vi "GPS (11.25).vi"() -> ()   [LabVIEW 2018]
uses:
  <vilib>/Instr/_visa.llb/VISA Configure Serial Port (Instr).vi
  <vilib>/Utility/file.llb/Read Delimited Spreadsheet (DBL).vi
panel:
  in  "로깅 정지":bool
  in  "Logging 저장위치":path
  in  "Logging On/Off":bool
  out "in out 상태":bool
  out "직선":bool
  out "곡선":bool
  out "주행완료":bool
  out "count":dbl
  out "설정 반지름":dbl
  out "중간":bool
  out "in":bool
  out "out":bool
  out "코스 판별":dbl(slide) scale=0.0..1.0
  out "out 근접":dbl
  out "in 근접":dbl
  out "RDDF Y_in":dbl[](array[numeric]) format="%#_10g"
  out "RDDF X_in":dbl[](array[numeric]) format="%#_10g"
  out "RDDF Y_out":dbl[](array[numeric]) format="%#_10g"
  out "RDDF X_out":dbl[](array[numeric]) format="%#_10g"
  in  "RDDF out 불러오기":path
  out "인터넷 지연 인덱스":u16
  out "최대 인터넷 지연속도":dbl
  out "목표속도(m/s)":dbl format="%#_13g"
  out "현재 인덱스":u16
  out "RDDF Y":dbl[](array[numeric]) format="%#_10g"
  out "RDDF X":dbl[](array[numeric]) format="%#_10g"
  out "Main Control 이상감지, Sub Control 전환":bool
  out "목표 Y":dbl format="%#_10g"
  out "목표 X":dbl format="%#_10g"
  in  "GPS신호읽기 정지버튼":bool
  in  "전체 정지":bool
  out "새로운 GPS데이터 획득":bool
  out "인터넷불량":bool
  in  "Dead Reckoning On":bool
  out "COG1":dbl
  out "속도2":dbl
  out "COG2":dbl
  out "COG 오차":dbl
  out "속도 오차":dbl
  in  "속도, cog 정지버튼":bool
  out "속도제한":bool
  out "목표 조향각":dbl(knob) scale=-20.0..20.0
  out "보정된 현재 Y":dbl format="%#.10g"
  out "보정된 현재 X":dbl format="%#.10g"
  in  "설정 속도":dbl
  in  "위치 데이터 보간 정지버튼":bool
  in  "Pure pursuit 정지버튼":bool
  out "속도1":dbl
  in  "목표 waypoint 정지버튼":bool
  in  "RDDF 불러오기 On/Off":bool
  in  "RDDF in 불러오기":path
  in  "경로 저장 On/Off":bool
  in  "현재 경로 저장위치":path
  out "XY 그래프":cluster{"all rows":dbl[], "all rows":dbl[]}[](graph)
  out "COG":dbl
  out "현재 Y":dbl format="%#.10g"
  out "현재 X":dbl format="%#.10g"
  out "GNRMC":string[](array[string])
  out "error out":errorcluster
  in  "baud rate (115200)":u32=115200 min=115200 max=115200
  in  "VISA resource name":refnum<visa-resource-name>
  # "in"
  # "out"
  # "주행 기록"
  # "시작 전 설정"
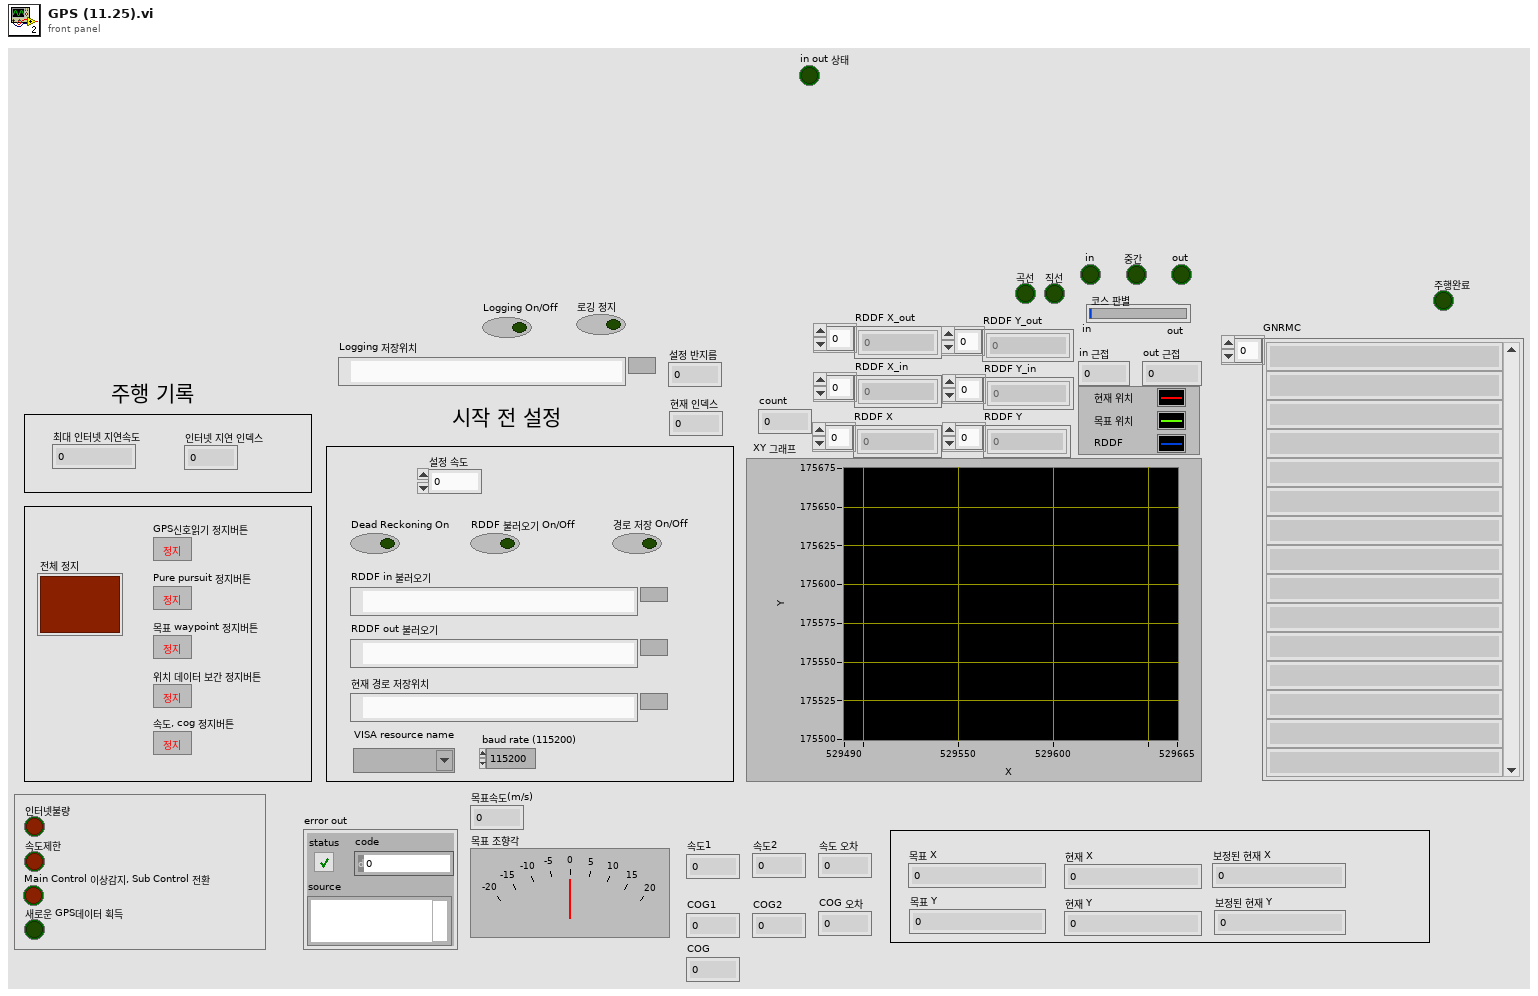
[diagram p1: front panel]
types:
  T1 = cluster{dbl, dbl, "left(2) 2":bool, "go and left(1) 2":bool, "left(2) 3":bool, "left(2) 4":bool, "left(2) 5":bool, "left(2) 6":bool, dbl}
  T2 = cluster{"목표 조향각":dbl, "목표속도(m/s)":dbl, bool, bool, "in":bool, "중간":bool, "out":bool, "주행완료":bool, "코스 판별":dbl}
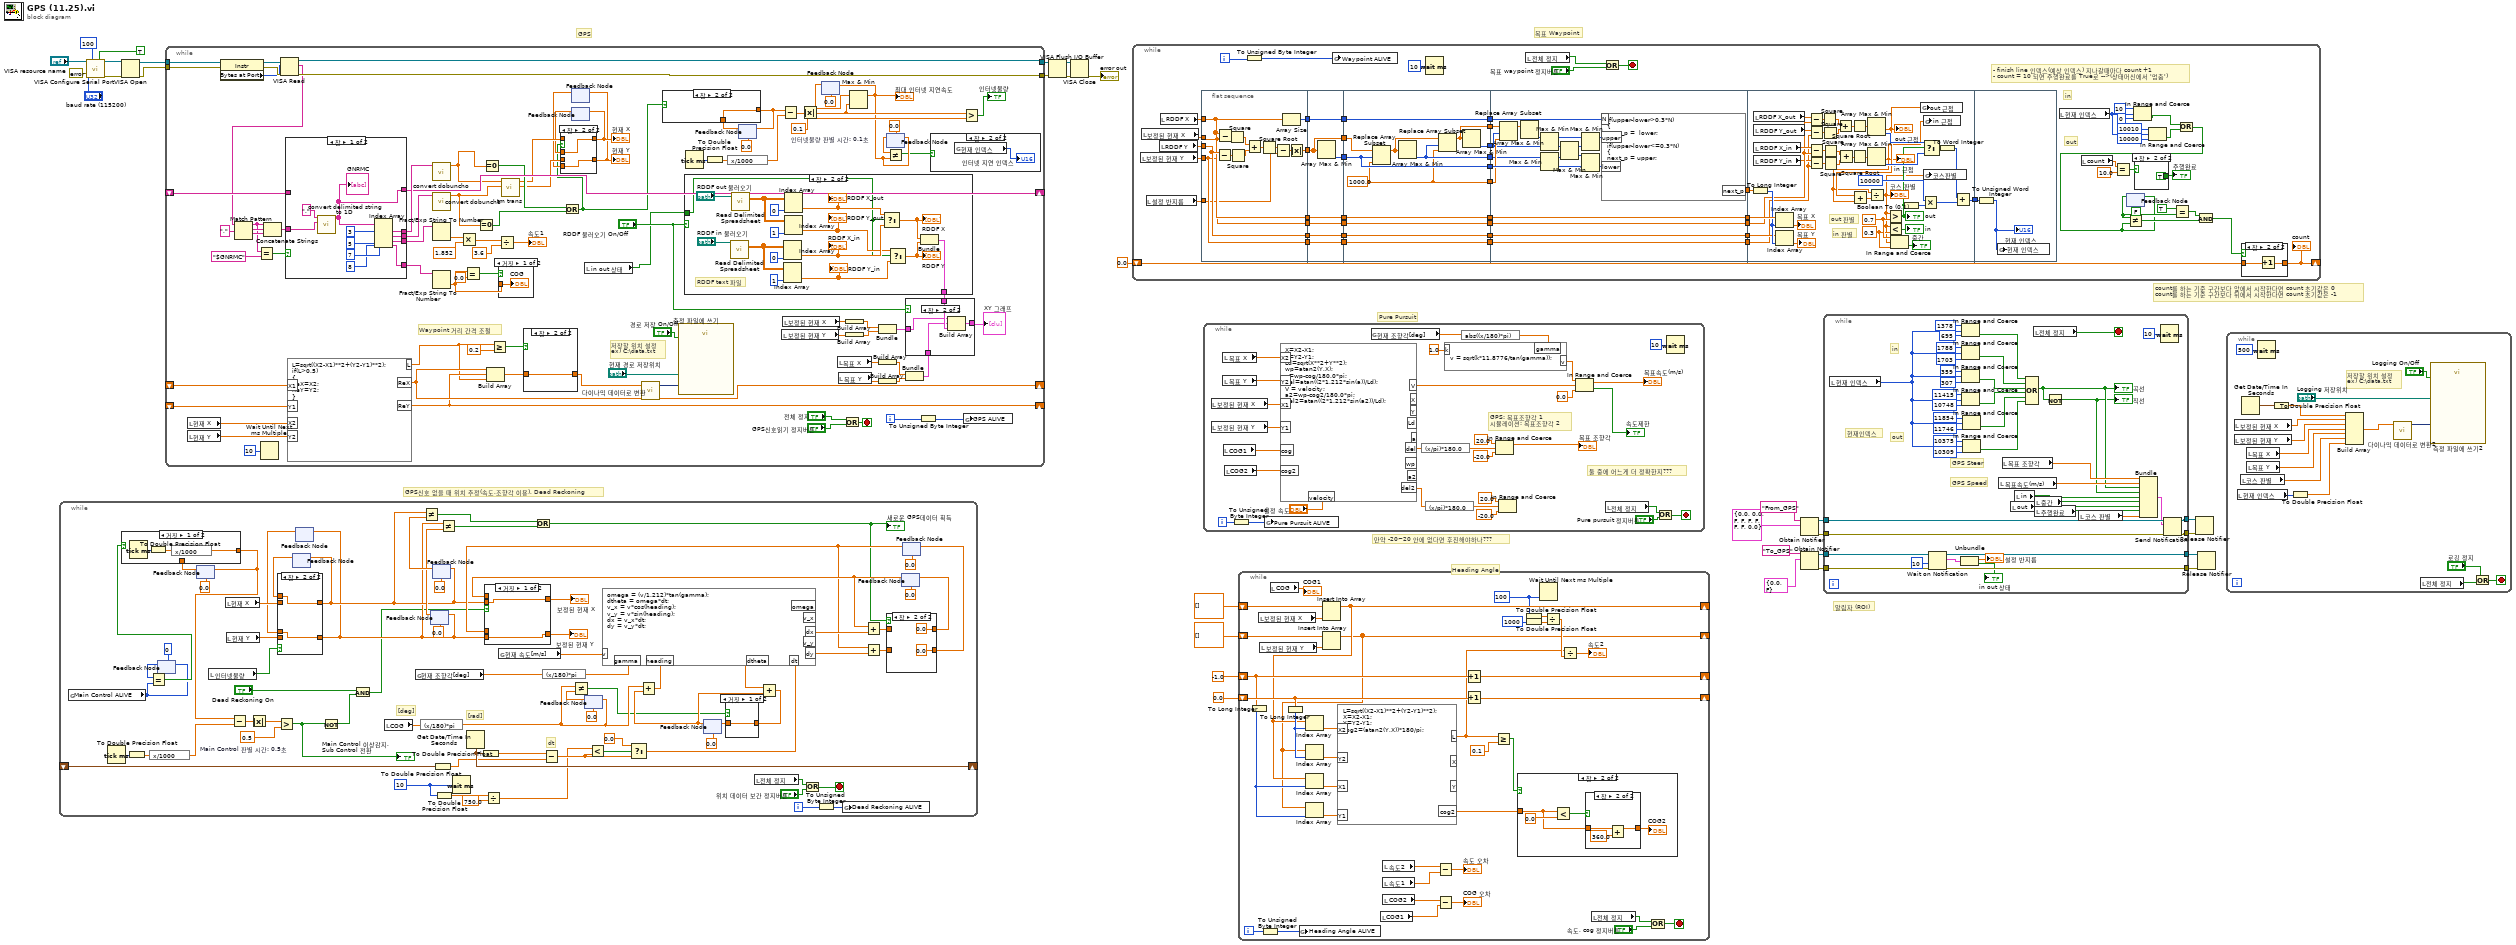
[diagram p0: block diagram]
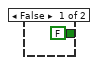
[diagram p3: hidden frame]
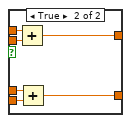
[diagram p8: hidden frame]
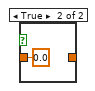
[diagram p9: hidden frame]
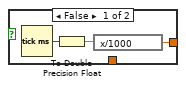
[diagram p12: hidden frame]
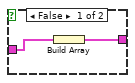
[diagram p14: hidden frame]
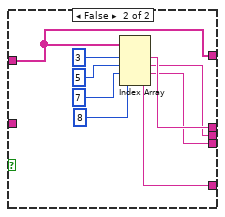
[diagram p18: hidden frame]
diagram:
  # "count를 하는 기준 구간보다 앞에서 시작한다면 count 초기값은 0\ncount를 하는 기준 구간보다 뒤에서 시작한다면 count 초기값은 -1"
  # "알림자 (ROI)"
  # "Heading Angle"
  # "Pure Pursuit"
  # "GPS"
  # "만약 -20~20 안에 없다면 후진해야하나???"
  # "GPS신호 없을 때 위치 추정(속도,조향각 이용), Dead Reckoning"
  # "목표 Waypoint"
  n1 = while {
    shift-right: [w104] -> _
    shift-left: _ -> [w105]
    i -> [w62]
    stop <- w52 stop-if-true
    w41 = 0.5  # Main Control 판별 시간: 0.5초
    w98 = u32 10 ("대기 시간 (ms)")
    # "[rad]"
    # "[deg]"
    # "dt"
    n2 = global read "글로벌 (11.23).vi" "Main Control ALIVE"() -> (w37:u8)
    n3 = Tick Count (ms)() -> (millisecond timer value=w48:u32)
    n4 = To Double Precision Float(number=w48) -> (double precision float=w38:dbl)
    n5 = expression code="x/1000"(w38) -> (w40:dbl)
    n6 = feedback #1(u8 0 ("Dead Reckoning ALIVE")) -> (w49:u8)
    n7 = Equal?(x=w49, y=w37) -> (x = y?=w43:bool)
    n8 = feedback-in #1(w37) -> ()
    n9 = feedback #2(0.0) -> (w47:dbl)
    n10 = case shown="거짓" w43 {
      tunnel: [w106 w109] -> w45
      tunnel: w47 -> [_ w109]
      frame False {
        n11 = Tick Count (ms)() -> (millisecond timer value=w107:u32)
        n12 = To Double Precision Float(number=w107) -> (double precision float=w108:dbl)
        n13 = expression code="x/1000"(w108) -> (w106:dbl)
      }
      frame True {
      }
    }
    n14 = feedback-in #2(w45) -> ()
    n15 = local read "인터넷불량"() -> (w53:bool)
    n16 = local read "현재 X"() -> (w59:dbl)
    n17 = local read "현재 Y"() -> (w58:dbl)
    n18 = Subtract(x=w45, y=w40) -> (x-y=w44:dbl)
    n19 = Absolute Value(x=w44) -> (abs(x)=w42:dbl)
    n20 = Greater?(x=w42, y=w41) -> (0:w36:bool)
    "Main Control 이상감지, Sub Control 전환" <- w36
    n21 = feedback #3() -> (w55:dbl)  [unwired: 1 in]
    n22 = feedback #4() -> (w54:dbl)  [unwired: 1 in]
    n23 = case shown="참" w53 {
      tunnel: [w111 w113] -> w57
      tunnel: w59 -> [w111 _]
      tunnel: [w110 w112] -> w56
      tunnel: w58 -> [w110 _]
      tunnel: w55 -> [_ w113]
      tunnel: w54 -> [_ w112]
      frame False {
      }
      frame True {
      }
    }
    n24 = feedback-in #3(w57) -> ()
    n25 = feedback-in #4(w56) -> ()
    n26 = Not(x=w36) -> (.not. x?=w35:bool)
    n27 = And(x="Dead Reckoning On", y=w35) -> (x .and. y?=w33:bool)
    n28 = local read "COG"() -> (w92:dbl)
    n29 = global read "글로벌 (11.23).vi" "현재 조향각[deg]"() -> (w32:dbl)
    n30 = expression code="(x/180)*pi"(w92) -> (w88:dbl)
    n31 = feedback #5(0.0 ("현재 Y")) -> (w72:dbl)
    n32 = feedback-in #5(w56) -> ()
    n33 = feedback #6(0.0 ("현재 X")) -> (w74:dbl)
    n34 = Not Equal?(x=w57, y=w74) -> (x != y?=w70:bool)
    n35 = feedback-in #6(w57) -> ()
    n36 = To Double Precision Float(number=w105) -> (double precision float=w103:dbl)
    n37 = To Double Precision Float(number=w98) -> (double precision float=w97:dbl)
    n38 = Not Equal?(x=w56, y=w72) -> (x != y?=w71:bool)
    n39 = Wait (ms)(milliseconds to wait=w98) -> ()  [unwired: 1 out]
    n40 = Get Date/Time In Seconds() -> (seconds since 1Jan1904=w104:timestamp)
    n41 = To Double Precision Float(number=w104) -> (double precision float=w102:dbl)
    n42 = Divide(x=w97, y=750.0) -> (x/y=w95:dbl)
    n43 = global read "글로벌 (11.23).vi" "현재 속도[m/s]"() -> (w65:dbl)
    n44 = Or(x=w70, y=w71) -> (x .or. y?=w67:bool)
    "새로운 GPS데이터 획득" <- w67
    n45 = expression code="(x/180)*pi"(w32) -> (w64:dbl)
    n46 = Subtract(x=w102, y=w103) -> (x-y=w99:dbl)
    n47 = feedback-in #7(w88) -> ()
    n48 = feedback #7(0.0 ("COG")) -> (w90:dbl)
    n49 = Not Equal?(x=w88, y=w90) -> (x != y?=w81:bool)
    n50 = Less?(x=w95, y=w99) -> (x < y?=w100:bool)
    n51 = Select(t=0.0, s=w100, f=w99) -> (s? t:f=w87:dbl)
    n52 = feedback #8(0.0) -> (w82:dbl)
    n53 = Add(x=w88, y=w82) -> (x+y=w89:dbl)
    n54 = formula code="omega = (v/1.212)*tan(gamma);\ndtheta = omega*dt;\nv_x = v*cos(heading);\nv_y = v*sin(heading);\ndx = v_x*dt;\ndy = v_y*dt;"("heading"=w89, "v"=w65, "dt"=w87, "gamma"=w64) -> ("dtheta"=w86:dbl, "dy"=w80:dbl, "dx"=w79:dbl)  [unwired: 3 out]
    n55 = local read "전체 정지"() -> (w51:bool)
    n56 = Add(x=w86, y=w82) -> (x+y=w85:dbl)
    n57 = case shown="거짓" w81 {
      tunnel: w85 -> [w122 _]
      tunnel: [w122 0.0] -> w84
      frame False {
      }
      frame True {
      }
    }
    n58 = feedback-in #8(w84) -> ()
    n59 = Or(x=w51, y="위치 데이터 보간 정지버튼") -> (x .or. y?=w52:bool)
    n60 = To Unsigned Byte Integer(number=w62) -> (unsigned 8bit integer=w63:u8)
    n61 = global write "글로벌 (11.23).vi" "Dead Reckoning ALIVE"(w63) -> ()
    n62 = feedback #9(0.0) -> (w69:dbl)
    n63 = Add(x=w69, y=w79) -> (x+y=w93:dbl)
    n64 = feedback #10(0.0) -> (w68:dbl)
    n65 = case shown="거짓" w33 {
      tunnel: w57 -> [w115 w121]
      tunnel: w56 -> [w114 w120]
      tunnel: w69 -> [_ w119]
      tunnel: w68 -> [_ w118]
      tunnel: [w115 w117] -> w61
      tunnel: [w114 w116] -> w60
      frame False {
      }
      frame True {
        n66 = Add(x=w119, y=w121) -> (x+y=w117:dbl)
        n67 = Add(x=w118, y=w120) -> (x+y=w116:dbl)
      }
    }
    "보정된 현재 X" <- w61
    "보정된 현재 Y" <- w60
    n68 = Add(x=w68, y=w80) -> (x+y=w94:dbl)
    n69 = case shown="참" w67 {
      tunnel: w94 -> [w125 _]
      tunnel: [w125 0.0] -> w77
      tunnel: w93 -> [w124 _]
      tunnel: [w124 0.0] -> w78
      frame False {
      }
      frame True {
      }
    }
    n70 = feedback-in #9(w78) -> ()
    n71 = feedback-in #10(w77) -> ()
  }
  n72 = call-poly "VISA Configure Serial Port"("VISA resource name"="VISA resource name", "timeout (10sec)"=u32 100, "Enable Termination\nChar (T)"=TRUE ("Enable Termination\nChar (T)"), "baud rate (9600)"="baud rate (115200)", "error in (no error)"=errorcluster {"status"=FALSE, "code"=0, "source"=""}) -> ("VISA resource name out"=w26:refnum<visa-resource-name>, "error out"=w27:errorcluster)  [unwired: 9 in]
  n73 = VISA Open(error in (no error)=w27, VISA resource name=w26) -> (VISA resource name=w24:refnum<visa-resource-name>, error out=w23:errorcluster)  [unwired: 3 in]
  n74 = while {
    tunnel: w24 -> [w217]
    tunnel: w23 -> [w216]
    tunnel: [w213] -> w19
    tunnel: [w212] -> w18
    shift-right: [w197] -> _
    shift-left: _ -> [w196]
    shift-right: [w190] -> _
    shift-left: _ -> [w192]
    shift-right: [w189] -> _
    shift-left: _ -> [w191]
    i -> [w172]
    stop <- w149 stop-if-true
    w155 = 0.1  # 인터넷불량 판별 시간: 0.1초
    # "Waypoint 거리 간격 조절"
    # "저장할 위치 설정\nex) C:\\data.txt"
    n75 = local read "현재 X"() -> (w194:dbl)
    n76 = local read "현재 Y"() -> (w193:dbl)
    n77 = property class="Instr"(reference=w217, error in=w216) -> (reference out=w215:refnum<visa-resource-name>, error out=w214:errorcluster, "Bytes at Port"=w211:u32)
    n78 = Wait Until Next ms Multiple(millisecond multiple=u32 10 ("ms 배수")) -> ()  [unwired: 1 out]
    n79 = VISA Read(VISA resource name=w215, byte count=w211, error in (no error)=w214) -> (VISA resource name out=w212:refnum<visa-resource-name>, read buffer=w129:string, error out=w213:errorcluster)  [unwired: 1 out]
    n80 = Match Pattern(string=w129, regular expression="," ("정규식")) -> (before substring=w199:string, match substring=w209:string, after substring=w208:string)  [unwired: 1 in, 1 out]
    n81 = Equal?(x=w199, y="$GNRMC" ("정규식")) -> (x = y?=w151:bool)
    n82 = Concatenate Strings(w199, w209, w208) -> (w207:string)
    n83 = case shown="참" w151 {
      tunnel: w207 -> [w257 _]
      tunnel: [w259 w266] -> w206
      tunnel: [w258 w265] -> w205
      tunnel: [w255 w264] -> w203
      tunnel: [w252 w263] -> w200
      tunnel: [w251 w262] -> w197
      tunnel: w196 -> [_ w262]
      frame True {
        n84 = call "convert delimited string to 1D.vi"("delimited string"=w257, "delimiter"=",") -> ("배열"=w251:string[])  [unwired: 9 in]
        "GNRMC" <- w251
        n85 = Index Array(array=w251, index #1=3 ("인덱스"), index #2=5 ("인덱스"), index #3=7 ("인덱스"), index #4=8 ("인덱스")) -> (element #1=w259:string, element #2=w258:string, element #3=w255:string, element #4=w252:string)
      }
      frame False {
        n86 = Index Array(array=w262, index #1=3 ("인덱스"), index #2=5 ("인덱스"), index #3=7 ("인덱스"), index #4=8 ("인덱스")) -> (element #1=w266:string, element #2=w265:string, element #3=w264:string, element #4=w263:string)
      }
    }
    n87 = formula code="L=sqrt((X2-X1)**2+(Y2-Y1)**2);\nif(L>0.5)\n{\nReX=X2;\nReY=Y2;\n}"("X2"=w194, "Y2"=w193, "X1"=w192, "Y1"=w191) -> ("ReX"=w190:dbl, "ReY"=w189:dbl, "L"=w188:dbl)
    n88 = call "convert dobuncho.vi"("GPS 데이터"=w206) -> ("숫자형"=w170:dbl)  [unwired: 10 in]
    n89 = call "convert dobuncho.vi"("GPS 데이터"=w205) -> ("숫자형"=w169:dbl)  [unwired: 10 in]
    n90 = Fract/Exp String To Number(string=w203) -> (number=w202:dbl)  [unwired: 3 in, 1 out]
    n91 = Fract/Exp String To Number(string=w200) -> (number=w176:dbl)  [unwired: 3 in, 1 out]
    n92 = Multiply(x=w202, y=1.852) -> (x*y=w179:dbl)
    n93 = Equal?(x=w176, y=0.0) -> (x = y?=w174:bool)
    n94 = Equal To 0?(x=w169) -> (x = 0?=w167:bool)
    n95 = Equal To 0?(x=w170) -> (x = 0?=w168:bool)
    n96 = Build Array(w190, w189, w188) -> (w185:dbl[])
    n97 = Greater Or Equal?(x=w188, y=0.2) -> (x >= y?=w186:bool)
    n98 = Divide(x=w179, y=3.6) -> (x/y=→"속도1":dbl)
    n99 = case shown="거짓" w174 {
      tunnel: w176 -> [w233 _]
      frame False {
        "COG" <- w233
      }
      frame True {
      }
    }
    n100 = call "tm trans.vi"("경도(Deg)"=w169, "위도(Deg)"=w170) -> ("E"=w165:dbl, "N"=w166:dbl)  [unwired: 8 in]
    n101 = case shown="참" w186 {
      tunnel: [_ w250] -> w184
      tunnel: w185 -> [_ w250]
      frame False {
      }
      frame True {
      }
    }
    n102 = Or(x=w168, y=w167) -> (x .or. y?=w152:bool)
    n103 = feedback #11() -> (w161:dbl)  [unwired: 1 in]
    n104 = feedback #12() -> (w162:dbl)  [unwired: 1 in]
    n105 = case shown="참" w152 {
      tunnel: w166 -> [w224 _]
      tunnel: [w224 w226] -> w164
      tunnel: [w223 w225] -> w163
      tunnel: w165 -> [w223 _]
      tunnel: w162 -> [_ w225]
      tunnel: w161 -> [_ w226]
      frame False {
      }
      frame True {
      }
    }
    "현재 X" <- w164
    "현재 Y" <- w163
    n106 = feedback-in #11(w164) -> ()
    n107 = feedback-in #12(w163) -> ()
    n108 = local read "in out 상태"() -> (w128:bool)
    n109 = call "다이나믹 데이터로 변환"("Array"=w184) -> ("Dynamic Data Type"=w183:dynamicdata)  [unwired: 3 in]
    n110 = call "측정 파일에 쓰기"("Signals"=w183, "Enable"="경로 저장 On/Off", "Filename"="현재 경로 저장위치") -> ()  [unwired: 14 in, 3 out]
    n111 = case shown="참" "RDDF 불러오기 On/Off" {
      tunnel: [_ w249] -> w180
      tunnel: w128 -> [_ w234]
      frame False {
      }
      frame True {
        # "RDDF text 파일"
        n112 = call-poly <vilib>:"Read Delimited Spreadsheet.vi"("file path (dialog if empty)"="RDDF in 불러오기") -> ("all rows"=w244:dbl[][])  [unwired: 9 in, 5 out]
        n113 = call-poly <vilib>:"Read Delimited Spreadsheet.vi"("file path (dialog if empty)"="RDDF out 불러오기") -> ("all rows"=w247:dbl[][])  [unwired: 9 in, 5 out]
        n114 = Index Array(array=w244, index (col)=0 ("비활성화된 인덱스 (열)")) -> (element=w238:dbl[])  [unwired: 1 in]
        "RDDF X_in" <- w238
        n115 = Index Array(array=w244, index (col)=1 ("비활성화된 인덱스 (열)")) -> (element=w236:dbl[])  [unwired: 1 in]
        "RDDF Y_in" <- w236
        n116 = Index Array(array=w247, index (col)=0 ("비활성화된 인덱스 (열)")) -> (element=w239:dbl[])  [unwired: 1 in]
        "RDDF X_out" <- w239
        n117 = Index Array(array=w247, index (col)=1 ("비활성화된 인덱스 (열)")) -> (element=w237:dbl[])  [unwired: 1 in]
        "RDDF Y_out" <- w237
        n118 = Select(t=w239, s=w234, f=w238) -> (s? t:f=w240:dbl[])
        "RDDF X" <- w240
        n119 = Select(t=w237, s=w234, f=w236) -> (s? t:f=w235:dbl[])
        "RDDF Y" <- w235
        n120 = Bundle("all rows"=w240, "all rows"=w235) -> (w249:cluster{"all rows":dbl[], "all rows":dbl[]})  [unwired: 1 in]
      }
    }
    n121 = Tick Count (ms)() -> (millisecond timer value=w160:u32)
    n122 = To Double Precision Float(number=w160) -> (double precision float=w153:dbl)
    n123 = expression code="x/1000"(w153) -> (w154:dbl)
    n124 = feedback #13(0.0) -> (w159:dbl)
    n125 = case shown="참" w152 {
      tunnel: [w219 w222] -> w157
      tunnel: w159 -> [_ w222]
      frame False {
        n126 = Tick Count (ms)() -> (millisecond timer value=w220:u32)
        n127 = To Double Precision Float(number=w220) -> (double precision float=w221:dbl)
        n128 = expression code="x/1000"(w221) -> (w219:dbl)
      }
      frame True {
      }
    }
    n129 = feedback-in #13(w157) -> ()
    n130 = Subtract(x=w157, y=w154) -> (x-y=w156:dbl)
    n131 = local read "보정된 현재 Y"() -> (w141:dbl)
    n132 = local read "보정된 현재 X"() -> (w140:dbl)
    n133 = Absolute Value(x=w156) -> (abs(x)=w135:dbl)
    n134 = feedback #14(0.0) -> (w134:dbl)
    n135 = local read "목표 X"() -> (w144:dbl)
    n136 = local read "목표 Y"() -> (w146:dbl)
    n137 = Or(x="전체 정지", y="GPS신호읽기 정지버튼") -> (x .or. y?=w149:bool)
    n138 = Build Array(w140) -> (w139:dbl[])
    n139 = Build Array(w141) -> (w138:dbl[])
    n140 = Max & Min(x=w134, y=w135) -> (max(x,y)=w131:dbl)  [unwired: 1 out]
    "최대 인터넷 지연속도" <- w131
    n141 = feedback-in #14(w131) -> ()
    n142 = Build Array(w144) -> (w143:dbl[])
    n143 = Build Array(w146) -> (w145:dbl[])
    n144 = Bundle(w139, w138) -> (w137:cluster{dbl[], dbl[]})  [unwired: 1 in]
    n145 = feedback #15(0.0 ("주행중 최대속도[m/s]")) -> (w133:dbl)
    n146 = feedback-in #15(w131) -> ()
    n147 = Not Equal?(x=w133, y=w131) -> (x != y?=w130:bool)
    n148 = Bundle(w143, w145) -> (w142:cluster{dbl[], dbl[]})  [unwired: 1 in]
    n149 = case shown="참" "RDDF 불러오기 On/Off" {
      tunnel: [w228 w232] -> w181
      tunnel: w180 -> [_ w231]
      tunnel: w142 -> [_ w230]
      tunnel: w137 -> [w227 w229]
      frame False {
        n150 = Build Array(w227) -> (w228:cluster{dbl[], dbl[]}[])
      }
      frame True {
        n151 = Build Array(w229, w230, w231) -> (w232:cluster{"all rows":dbl[], "all rows":dbl[]}[])
      }
    }
    "XY 그래프" <- w181
    n152 = To Unsigned Byte Integer(number=w172) -> (unsigned 8bit integer=w171:u8)
    n153 = case shown="참" w130 {
      frame False {
      }
      frame True {
        n154 = global read "글로벌 (11.23).vi" "현재 인덱스"() -> (→"인터넷 지연 인덱스":u16)
      }
    }
    n155 = Greater?(x=w135, y=w155) -> (0:→"인터넷불량":bool)
    n156 = global write "글로벌 (11.23).vi" "GPS ALIVE"(w171) -> ()
  }
  n157 = VISA Flush I/O Buffer(VISA resource name=w18, error in (no error)=w19) -> (VISA resource name out=w21:refnum<visa-resource-name>, error out=w22:errorcluster)  [unwired: 1 in]
  n158 = VISA Close(VISA resource name=w21, error in (no error)=w22) -> (error out=→"error out":errorcluster)
  n159 = while {
    shift-right: [w286] -> _
    shift-left: 0.0 -> [w285]
    i -> [w325]
    stop <- w326 stop-if-true
    # "in"
    # "out"
    # "- finish line 인덱스(예상 인덱스) 지나갈때마다 count +1\n- count = 10 되면 주행완료를 True로 -->(상태머신에서 '멈춤')"
    n160 = local read "보정된 현재 Y"() -> (w302:dbl)
    n161 = local read "보정된 현재 X"() -> (w300:dbl)
    n162 = local read "설정 반지름"() -> (w303:dbl)
    n163 = local read "RDDF Y"() -> (w324:dbl[])
    n164 = local read "RDDF X"() -> (w301:dbl[])
    n165 = flat-sequence {
      tunnel: w301 -> [w342]
      tunnel: w324 -> [w349]
      tunnel: w300 -> [w338]
      tunnel: w302 -> [w337]
      tunnel: w303 -> [w336]
      tunnel: [w340] -> w323
      tunnel: [w339] -> w319
      tunnel: [w342] -> w318
      tunnel: [w349] -> w317
      tunnel: [w338] -> w299
      tunnel: [w337] -> w298
      tunnel: w323 -> [w355]
      tunnel: [w356] -> w322
      tunnel: [w355] -> w321
      tunnel: [w354] -> w320
      tunnel: w319 -> [w354]
      tunnel: w318 -> [w353]
      tunnel: w317 -> [w352]
      tunnel: [w353] -> w316
      tunnel: [w352] -> w315
      tunnel: w299 -> [w351]
      tunnel: w298 -> [w350]
      tunnel: [w351] -> w295
      tunnel: [w350] -> w292
      tunnel: w322 -> [w364]
      tunnel: w321 -> [w368]
      tunnel: w320 -> [w365]
      tunnel: [w367] -> w314
      tunnel: w316 -> [w367]
      tunnel: [w366] -> w312
      tunnel: w315 -> [w366]
      tunnel: [w365] -> w309
      tunnel: [w364] -> w308
      tunnel: [w362] -> w307
      tunnel: [w361] -> w306
      tunnel: [w360] -> w305
      tunnel: [w359] -> w304
      tunnel: [w358] -> w296
      tunnel: w295 -> [w358]
      tunnel: [w357] -> w293
      tunnel: w292 -> [w357]
      tunnel: w314 -> [w389]
      tunnel: [w389] -> w313
      tunnel: w312 -> [w388]
      tunnel: [w388] -> w311
      tunnel: [w387] -> w310
      tunnel: w309 -> [w372]
      tunnel: w308 -> [w386]
      tunnel: w307 -> [w379]
      tunnel: w306 -> [w380]
      tunnel: w305 -> [w384]
      tunnel: w304 -> [w383]
      tunnel: [w370] -> w297
      tunnel: w296 -> [w370]
      tunnel: [w369] -> w294
      tunnel: w293 -> [w369]
      tunnel: w313 -> [w430]
      tunnel: w311 -> [w425]
      tunnel: w310 -> [w429]
      tunnel: w297 -> [w416]
      tunnel: w294 -> [w414]
      tunnel: [w399] -> w291
      tunnel: w291 -> [w431]
      frame #0 {
        n166 = Subtract(x=w349, y=w337) -> (x-y=w347:dbl[])
        n167 = Subtract(x=w342, y=w338) -> (x-y=w348:dbl[])
        n168 = Square(x=w348) -> (x^2=w346:dbl[])
        n169 = Square(x=w347) -> (x^2=w345:dbl[])
        n170 = Add(x=w346, y=w345) -> (x+y=w344:dbl[])
        n171 = Square Root(x=w344) -> (sqrt(x)=w343:dbl[])
        n172 = Subtract(x=w343, y=w336) -> (x-y=w341:dbl[])
        n173 = Array Size(array=w342) -> (size(s)=w339:i32)
        n174 = Absolute Value(x=w341) -> (abs(x)=w340:dbl[])
      }
      frame #1 {
        n175 = Array Max & Min(array=w355) -> (min index (indices)=w356:i32)  [unwired: 3 out]
      }
      frame #2 {
        w359 = 1000.0 ("새 원소/부분배열")
        n176 = Replace Array Subset(array=w368, new element=w359, index=w364) -> (w363:dbl[])
        n177 = Array Max & Min(array=w363) -> (min index (indices)=w362:i32)  [unwired: 3 out]
        n178 = Replace Array Subset(array=w363, new element=w359, index=w362) -> (w360:dbl[])
        n179 = Array Max & Min(array=w360) -> (min index (indices)=w361:i32)  [unwired: 3 out]
      }
      frame #3 {
        n180 = Replace Array Subset(array=w384, new element=w383, index=w380) -> (w382:dbl[])
        n181 = Array Max & Min(array=w382) -> (min index (indices)=w381:i32)  [unwired: 3 out]
        n182 = Max & Min(x=w381, y=w380) -> (max(x,y)=w375:i32, min(x,y)=w378:i32)
        n183 = Max & Min(x=w379, y=w386) -> (max(x,y)=w385:i32, min(x,y)=w377:i32)
        n184 = Max & Min(x=w378, y=w385) -> (max(x,y)=w374:i32, min(x,y)=w376:i32)
        n185 = Max & Min(x=w375, y=w374) -> (max(x,y)=w371:i32)  [unwired: 1 out]
        n186 = Max & Min(x=w376, y=w377) -> (min(x,y)=w373:i32)  [unwired: 1 out]
        n187 = formula code="if(upper-lower>0.3*N)\n{\nnext_p =  lower;\n}\nif(upper-lower<=0.3*N)\n{\nnext_p = upper;\n}"("N"=w372, "upper"=w371, "lower"=w373) -> ("next_p"=w387:dbl)
      }
      frame #4 {
        w404 = 0.3 ("y")
        w405 = 0.7 ("y")
        # "in 판별"
        # "out 판별"
        n188 = To Long Integer(number=w429) -> (32bit integer=w426:i32)
        n189 = local read "RDDF X_out"() -> (w424:dbl[])
        n190 = local read "RDDF Y_out"() -> (w422:dbl[])
        n191 = local read "RDDF X_in"() -> (w417:dbl[])
        n192 = local read "RDDF Y_in"() -> (w415:dbl[])
        n193 = Index Array(array=w430, index=w426) -> (element=→"목표 X":dbl)
        n194 = Index Array(array=w425, index=w426) -> (element=→"목표 Y":dbl)
        n195 = Subtract(x=w424, y=w416) -> (x-y=w423:dbl[])
        n196 = Subtract(x=w422, y=w414) -> (x-y=w421:dbl[])
        n197 = Subtract(x=w417, y=w416) -> (x-y=w413:dbl[])
        n198 = Subtract(x=w415, y=w414) -> (x-y=w412:dbl[])
        n199 = Square(x=w423) -> (x^2=w419:dbl[])
        n200 = Square(x=w421) -> (x^2=w420:dbl[])
        n201 = Square(x=w413) -> (x^2=w411:dbl[])
        n202 = Square(x=w412) -> (x^2=w410:dbl[])
        n203 = Add(x=w419, y=w420) -> (x+y=w418:dbl[])
        n204 = Add(x=w411, y=w410) -> (x+y=w409:dbl[])
        n205 = Square Root(x=w418) -> (sqrt(x)=w408:dbl[])
        n206 = Square Root(x=w409) -> (sqrt(x)=w407:dbl[])
        n207 = Array Max & Min(array=w408) -> (min value=w391:dbl, min index (indices)=w398:i32)  [unwired: 2 out]
        "out 근접" <- w391
        n208 = Array Max & Min(array=w407) -> (min value=w390:dbl, min index (indices)=w397:i32)  [unwired: 2 out]
        "in 근접" <- w390
        n209 = Add(x=w391, y=w390) -> (x+y=w406:dbl)
        n210 = Divide(x=w390, y=w406) -> (x/y=w392:dbl)
        "코스 판별" <- w392
        n211 = Greater?(x=w392, y=w405) -> (0:w393:bool)
        "out" <- w393
        n212 = Less?(x=w392, y=w404) -> (x < y?=→"in":bool)
        n213 = In Range and Coerce(upper limit=w405, x=w392, lower limit=w404) -> (In Range?=→"중간":bool)  [unwired: 1 out]
        n214 = Boolean To (0,1)(Boolean=w393) -> (0, 1=w401:i16)
        n215 = global write "글로벌 (11.23).vi" "out 근접"(w391) -> ()
        n216 = Multiply(x=i16 10000, y=w401) -> (x*y=w396:i16)
        n217 = Select(t=w398, s=w393, f=w397) -> (s? t:f=w394:i32)
        n218 = global write "글로벌 (11.23).vi" "in 근접"(w390) -> ()
        n219 = global write "글로벌 (11.23).vi" "코스판별"(w392) -> ()
        n220 = To Word Integer(number=w394) -> (16bit integer=w395:i16)
        n221 = Add(x=w395, y=w396) -> (x+y=w399:i16)
      }
      frame #5 {
        n222 = To Unsigned Word Integer(number=w431) -> (unsigned 16bit integer=w432:u16)
        "현재 인덱스" <- w432
        n223 = global write "글로벌 (11.23).vi" "현재 인덱스"(w432) -> ()
      }
    }
    n224 = To Unsigned Byte Integer(number=w325) -> (unsigned 8bit integer=w330:u8)
    n225 = global write "글로벌 (11.23).vi" "Waypoint ALIVE"(w330) -> ()
    n226 = Wait (ms)(milliseconds to wait=u32 10 ("대기 시간 (ms)")) -> ()  [unwired: 1 out]
    n227 = local read "전체 정지"() -> (w328:bool)
    n228 = Or(x=w328, y="목표 waypoint 정지버튼") -> (x .or. y?=w326:bool)
    n229 = local read "현재 인덱스"() -> (w277:u16)
    n230 = local read "count"() -> (w288:dbl)
    n231 = Equal?(x=w288, y=10.0) -> (x = y?=w290:bool)
    n232 = feedback #16(FALSE) -> (w280:bool)
    n233 = In Range and Coerce(upper limit=u16 10 ("하위 리미트"), x=w277, lower limit=u16 0 ("하위 리미트")) -> (In Range?=w273:bool)  [unwired: 1 out]
    n234 = case shown="참" w290 {
      tunnel: [FALSE TRUE] -> w287
      frame False {
      }
      frame True {
      }
    }
    "주행완료" <- w287
    n235 = In Range and Coerce(upper limit=u16 10010 ("상위 리미트"), x=w277, lower limit=u16 10000 ("하위 리미트")) -> (In Range?=w274:bool)  [unwired: 1 out]
    n236 = Equal?(x=TRUE, y=w280) -> (x = y?=w279:bool)
    n237 = Or(x=w273, y=w274) -> (x .or. y?=w272:bool)
    n238 = feedback-in #16(w272) -> ()
    n239 = Not Equal?(x=w280, y=w272) -> (x != y?=w282:bool)
    n240 = And(x=w279, y=w282) -> (x .and. y?=w278:bool)
    n241 = case shown="참" w278 {
      tunnel: [w331 w333] -> w286
      tunnel: w285 -> [w331 w332]
      frame False {
      }
      frame True {
        n242 = Increment(x=w332) -> (x+1=w333:dbl)
      }
    }
    "count" <- w286
  }
  n243 = while {
    i -> [w438]
    stop <- w435 stop-if-true
    # "GPS: 목표조향각 1\n시뮬레이션: 목표조향각 2"
    # "둘 중에 어느게 더 정확한지???"
    n244 = local read "보정된 현재 X"() -> (w455:dbl)
    n245 = local read "보정된 현재 Y"() -> (w456:dbl)
    n246 = local read "목표 X"() -> (w458:dbl)
    n247 = local read "목표 Y"() -> (w454:dbl)
    n248 = local read "COG1"() -> (w457:dbl)
    n249 = local read "COG2"() -> (w445:dbl)
    n250 = To Unsigned Byte Integer(number=w438) -> (unsigned 8bit integer=w439:u8)
    n251 = global write "글로벌 (11.23).vi" "Pure Pursuit ALIVE"(w439) -> ()
    n252 = formula code="X=X2-X1;\nY=Y2-Y1;\nLd=sqrt(X**2+Y**2);\nwp=atan2(Y,X);\na=wp-cog/180.0*pi;\ndel=atan((2*1.212*sin(a))/Ld);\nV = velocity;\na2=wp-cog2/180.0*pi;\ndel2=atan((2*1.212*sin(a2))/Ld);"("X2"=w458, "Y2"=w454, "X1"=w455, "Y1"=w456, "cog"=w457, "velocity"="설정 속도", "cog2"=w445) -> ("del"=w459:dbl, "V"=w451:dbl, "del2"=w441:dbl)  [unwired: 6 out]
    n253 = global read "글로벌 (11.23).vi" "현재 조향각[deg]"() -> (w449:dbl)
    n254 = expression code="(x/pi)*180.0"(w459) -> (w462:dbl)
    n255 = expression code="(x/pi)*180.0"(w441) -> (w442:dbl)
    n256 = expression code="abs((x/180)*pi)"(w449) -> (w448:dbl)
    n257 = formula code="v = sqrt(k*11.8776/tan(gamma));"("gamma"=w448, "k"=1.0 ("입력 변수")) -> ("v"=w450:dbl)
    n258 = In Range and Coerce(upper limit=20.0 ("상위 리미트"), x=w462, lower limit=-20.0 ("하위 리미트")) -> (coerced(x)=→"목표 조향각":dbl)  [unwired: 1 out]
    n259 = In Range and Coerce(upper limit=20.0 ("상위 리미트"), x=w442, lower limit=-20.0 ("하위 리미트")) -> ()  [unwired: 2 out]
    n260 = In Range and Coerce(upper limit=w450, x=w451, lower limit=0.0 ("하위 리미트")) -> (coerced(x)=→"목표속도(m/s)":dbl, In Range?=→"속도제한":bool)
    n261 = local read "전체 정지"() -> (w437:bool)
    n262 = Or(x=w437, y="Pure pursuit 정지버튼") -> (x .or. y?=w435:bool)
    n263 = Wait (ms)(milliseconds to wait=u32 10 ("대기 시간 (ms)")) -> ()  [unwired: 1 out]
  }
  n264 = while {
    shift-right: [w465] -> _
    shift-left: dbl[] [] -> [w498]
    shift-right: [w464] -> _
    shift-left: dbl[] [] -> [w497]
    shift-right: [w496] -> _
    shift-left: -1.0 -> [w492]
    shift-right: [w495] -> _
    shift-left: 0.0 -> [w494]
    i -> [w471]
    stop <- w468 stop-if-true
    w463 = u32 100 ("ms 배수")
    n265 = To Long Integer(number=w492) -> (32bit integer=w491:i32)
    n266 = local read "보정된 현재 X"() -> (w500:dbl)
    n267 = local read "보정된 현재 Y"() -> (w499:dbl)
    n268 = To Unsigned Byte Integer(number=w471) -> (unsigned 8bit integer=w472:u8)
    n269 = local read "COG"() -> (→"COG1":dbl)
    n270 = To Long Integer(number=w494) -> (32bit integer=w493:i32)
    n271 = global write "글로벌 (11.23).vi" "Heading Angle ALIVE"(w472) -> ()
    n272 = Insert Into Array(array=w498, new element=w500) -> (w465:dbl[])  [unwired: 1 in]
    n273 = Index Array(array=w465, index=w493) -> (element=w490:dbl)
    n274 = Index Array(array=w465, index=w491) -> (element=w487:dbl)
    n275 = Insert Into Array(array=w497, new element=w499) -> (w464:dbl[])  [unwired: 1 in]
    n276 = Index Array(array=w464, index=w493) -> (element=w488:dbl)
    n277 = Index Array(array=w464, index=w491) -> (element=w489:dbl)
    n278 = formula code="L=sqrt((X2-X1)**2+(Y2-Y1)**2);\nX=X2-X1;\nY=Y2-Y1;\ncog2=(atan2(Y,X))*180/pi;"("X2"=w490, "Y2"=w488, "X1"=w487, "Y1"=w489) -> ("L"=w475:dbl, "cog2"=w485:dbl)  [unwired: 2 out]
    n279 = local read "COG1"() -> (w480:dbl)
    n280 = local read "속도2"() -> (w483:dbl)
    n281 = local read "속도1"() -> (w482:dbl)
    n282 = local read "COG2"() -> (w481:dbl)
    n283 = Subtract(x=w483, y=w482) -> (x-y=→"속도 오차":dbl)
    n284 = Subtract(x=w481, y=w480) -> (x-y=→"COG 오차":dbl)
    n285 = Increment(x=w492) -> (x+1=w496:dbl)
    n286 = Increment(x=w494) -> (x+1=w495:dbl)
    n287 = Greater Or Equal?(x=w475, y=0.1) -> (x >= y?=w484:bool)
    n288 = case shown="참" w484 {
      tunnel: w485 -> [_ w502]
      frame False {
      }
      frame True {
        n289 = Less?(x=w502, y=0.0) -> (x < y?=w503:bool)
        n290 = case shown="참" w503 {
          tunnel: w502 -> [w505 w508]
          tunnel: [w505 w506] -> w501
          frame False {
          }
          frame True {
            n291 = Add(x=w508, y=360.0) -> (x+y=w506:dbl)
          }
        }
        "COG2" <- w501
      }
    }
    n292 = To Double Precision Float(number=w463) -> (double precision float=w467:dbl)
    n293 = To Double Precision Float(number=u32 1000 ("y")) -> (double precision float=w466:dbl)
    n294 = Wait Until Next ms Multiple(millisecond multiple=w463) -> ()  [unwired: 1 out]
    n295 = Divide(x=w467, y=w466) -> (x/y=w476:dbl)
    n296 = Divide(x=w475, y=w476) -> (x/y=→"속도2":dbl)
    n297 = local read "전체 정지"() -> (w470:bool)
    n298 = Or(x=w470, y="속도, cog 정지버튼") -> (x .or. y?=w468:bool)
  }
  n299 = Obtain Notifier(name (unnamed)="From_GPS" ("이름(이름없음)"), notification data type=T1 {0.0, 0.0, "left(2) 2"=FALSE, "go and left(1) 2"=FALSE, "left(2) 3"=FALSE, "left(2) 4"=FALSE, "left(2) 5"=FALSE, "left(2) 6"=FALSE, 0.0}) -> (notifier out=w10:refnum<notifier>, error out=w11:errorcluster)  [unwired: 2 in, 1 out]
  n300 = Obtain Notifier(name (unnamed)="To_GPS" ("이름(이름없음)"), notification data type=cluster{dbl, "left(2) 3":bool} {0.0, "left(2) 3"=FALSE}) -> (notifier out=w5:refnum<notifier>, error out=w4:errorcluster)  [unwired: 2 in, 1 out]
  n301 = while {
    tunnel: w10 -> [w551]
    tunnel: w11 -> [w550]
    tunnel: [w549] -> w12
    tunnel: [w548] -> w13
    tunnel: w5 -> [w541]
    tunnel: w4 -> [w540]
    tunnel: [w539] -> w3
    tunnel: [w538] -> w2
    stop <- w536 stop-if-true
    # "in"
    # "out"
    # "GPS Speed"
    # "GPS Steer"
    # "현재인덱스"
    n302 = local read "현재 인덱스"() -> (w525:u16)
    n303 = Wait on Notification(notifier=w541, timeout in ms (-1)=10 ("타임아웃(ms) (-1)"), error in (no error)=w540) -> (notifier out=w539:refnum<notifier>, notification=w543:cluster{dbl, "left(2) 3":bool}, error out=w538:errorcluster)  [unwired: 1 in, 1 out]
    n304 = Unbundle(w543) -> (→"설정 반지름":dbl, "left(2) 3"=→"in out 상태":bool)
    n305 = In Range and Coerce(upper limit=u16 1378 ("상위 리미트"), x=w525, lower limit=u16 695 ("하위 리미트")) -> (In Range?=w522:bool)  [unwired: 1 out]
    n306 = In Range and Coerce(upper limit=u16 1788 ("상위 리미트"), x=w525, lower limit=u16 1703 ("하위 리미트")) -> (In Range?=w521:bool)  [unwired: 1 out]
    n307 = In Range and Coerce(upper limit=u16 359 ("상위 리미트"), x=w525, lower limit=u16 307 ("하위 리미트")) -> (In Range?=w520:bool)  [unwired: 1 out]
    n308 = In Range and Coerce(upper limit=u16 11415 ("상위 리미트"), x=w525, lower limit=u16 10748 ("하위 리미트")) -> (In Range?=w519:bool)  [unwired: 1 out]
    n309 = In Range and Coerce(upper limit=u16 11854 ("상위 리미트"), x=w525, lower limit=u16 11746 ("하위 리미트")) -> (In Range?=w518:bool)  [unwired: 1 out]
    n310 = In Range and Coerce(upper limit=u16 10375 ("상위 리미트"), x=w525, lower limit=u16 10309 ("하위 리미트")) -> (In Range?=w517:bool)  [unwired: 1 out]
    n311 = local read "목표속도(m/s)"() -> (w546:dbl)
    n312 = local read "목표 조향각"() -> (w547:dbl)
    n313 = local read "out"() -> (w512:bool)
    n314 = local read "in"() -> (w514:bool)
    n315 = Compound Arithmetic op=OR ("복합 연산")(w522, w521, w520, w519, w518, w517) -> (w516:bool)
    "곡선" <- w516
    n316 = local read "전체 정지"() -> (w536:bool)
    n317 = local read "중간"() -> (w513:bool)
    n318 = local read "주행완료"() -> (w511:bool)
    n319 = Not(x=w516) -> (.not. x?=w515:bool)
    "직선" <- w515
    n320 = local read "코스 판별"() -> (w509:dbl)
    n321 = Bundle("목표 조향각"=w547, "목표속도(m/s)"=w546, w516, w515, "in"=w514, "중간"=w513, "out"=w512, "주행완료"=w511, "코스 판별"=w509) -> (w545:T2)  [unwired: 1 in]
    n322 = Wait (ms)(milliseconds to wait=u32 10 ("대기 시간 (ms)")) -> ()  [unwired: 1 out]
    n323 = Send Notification(notification=w545, notifier=w551, error in (no error)=w550) -> (notifier out=w549:refnum<notifier>, error out=w548:errorcluster)
  }
  n324 = Release Notifier(notifier=w12, error in (no error)=w13) -> ()  [unwired: 1 in, 3 out]
  n325 = Release Notifier(notifier=w3, error in (no error)=w2) -> ()  [unwired: 1 in, 3 out]
  n326 = while {
    stop <- w553 stop-if-true
    # "저장할 위치 설정\nex) C:\\data.txt"
    n327 = local read "보정된 현재 X"() -> (w563:dbl)
    n328 = local read "보정된 현재 Y"() -> (w562:dbl)
    n329 = local read "현재 인덱스"() -> (w556:u16)
    n330 = local read "코스 판별"() -> (w557:dbl)
    n331 = Get Date/Time In Seconds() -> (seconds since 1Jan1904=w561:timestamp)
    n332 = local read "목표 X"() -> (w559:dbl)
    n333 = local read "목표 Y"() -> (w558:dbl)
    n334 = Wait (ms)(milliseconds to wait=u32 500 ("대기 시간 (ms)")) -> ()  [unwired: 1 out]
    n335 = To Double Precision Float(number=w561) -> (double precision float=w560:dbl)
    n336 = To Double Precision Float(number=w556) -> (double precision float=w555:dbl)
    n337 = Build Array(w560, w563, w562, w559, w558, w557, w555) -> (w564:dbl[])
    n338 = call "다이나믹 데이터로 변환2"("Array"=w564) -> ("Dynamic Data Type"=w567:dynamicdata)  [unwired: 3 in]
    n339 = local read "전체 정지"() -> (w554:bool)
    n340 = call "측정 파일에 쓰기2"("Signals"=w567, "Enable"="Logging On/Off", "Filename"="Logging 저장위치") -> ()  [unwired: 14 in, 3 out]
    n341 = Or(x="로깅 정지", y=w554) -> (x .or. y?=w553:bool)
  }
